vi "QE open.vi"() -> (0 "QE data":cluster{"Numeric":dbl, dbl}[](array[cluster]))   [LabVIEW 2019]
uses:
  <vilib>/Utility/file.llb/Read Delimited Spreadsheet (DBL).vi
panel:
  out "XY Graph":cluster{"X":dbl, "Y":dbl}[](graph)
  out "QE":dbl[](array[numeric])
  out "eV":dbl[](array[numeric])
  in  "file path for tab delimited QE text file":path=path "C:/Users/Spenser Burrows/Desktop/Work/Labview software for spectrometer/BEN QE Curve.txt"
  # "Find BEN QE Curve.txt on the machine that this vi is being run on, then right click on the file box, go to data operations, and make current value default"
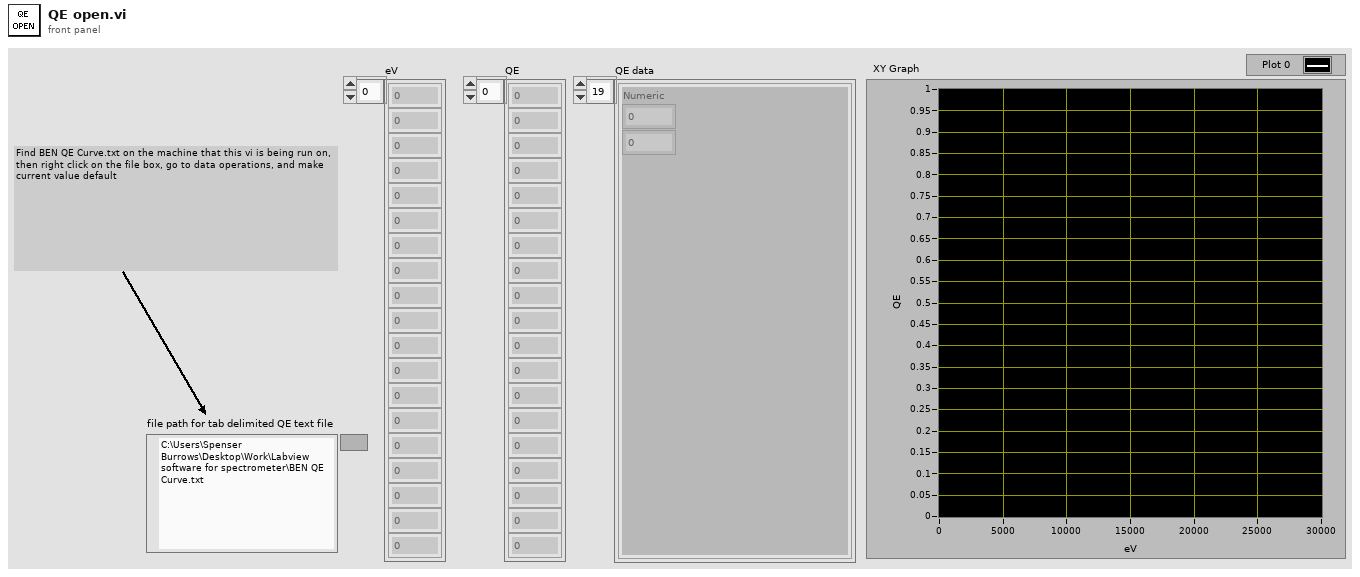
[diagram p1: front panel]
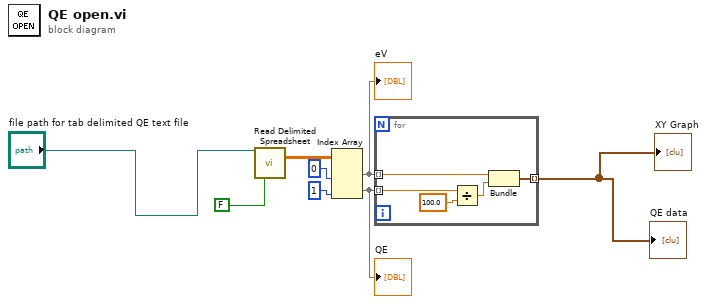
[diagram p0: block diagram]
diagram:
  n1 = call-poly <vilib>:"Read Delimited Spreadsheet.vi"("file path (dialog if empty)"="file path for tab delimited QE text file", "transpose? (F)"=FALSE) -> ("all rows"=w5:dbl[][])  [unwired: 8 in, 5 out]
  n2 = Index Array(array=w5, index (col) #1=0 ("disabled index (col)"), index (col) #2=1 ("disabled index (col)")) -> (element #1=w4:dbl[], element #2=w3:dbl[])  [unwired: 2 in]
  "eV" <- w4
  "QE" <- w3
  n3 = for {
    tunnel: w4 -> [w13] mode=indexing
    tunnel: w3 -> [w11] mode=indexing
    tunnel: [w12] -> w1 mode=indexing
    n4 = Divide(x=w11, y=100.0) -> (x/y=w9:dbl)
    n5 = Bundle("Numeric"=w13, w9) -> (w12:cluster{"Numeric":dbl, dbl})  [unwired: 1 in]
  }
  "QE data" <- w1
  "XY Graph" <- w1
